vi "Read triangles from stl file (binary format).vi"(0 "STL file path":path=path "C:/EnFlo Software/Anemometry/Anemometry Sub Vis/Collision_Detection/Triangles/Example files/SR-71_Blackbird.STL") -> (1 "Triangles array":T1[](array[typedef]), 2 "N triangles":u32=3528, 3 "Error out":errorcluster)   [LabVIEW 2014]
doc: "Note: The STL file must be in binary format, not ASCII."
uses:
  Typedefs/Triangle.ctl
panel:
  out "STL header":string
  # "PN 19/01/2015"
  # "Vertices"
  # "Edges"
  # "Unit normal"
  # "pre-store"
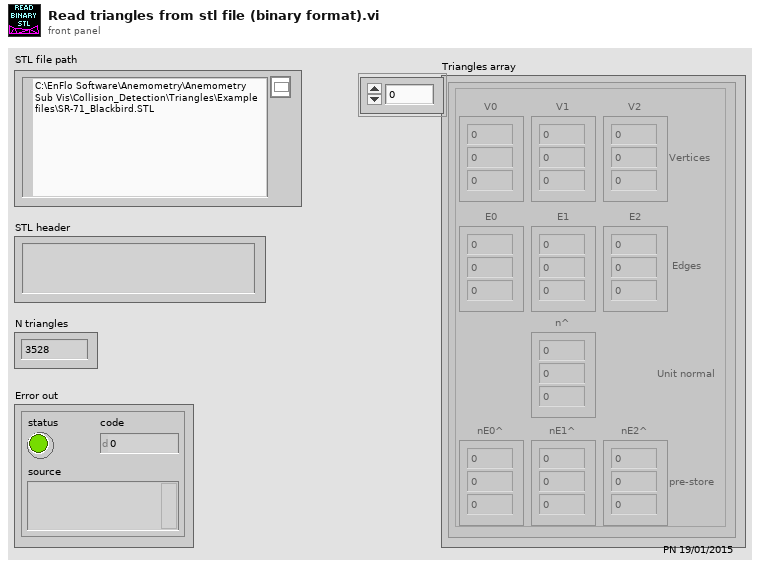
[diagram p1: front panel]
types:
  T1 = typedef "Triangle.ctl" = cluster{"V0":sgl[], "V1":sgl[], "V2":sgl[], "E0":sgl[], "E1":sgl[], "E2":sgl[], "n^":sgl[], "nE0^":sgl[], "nE1^":sgl[], "nE2^":sgl[]}
  T2 = enum16{"big-endian, network order", "native, host order", "little-endian"}
  T3 = enum16{"open", "replace", "create", "open or create", "replace or create", "replace or create with confirmation"}
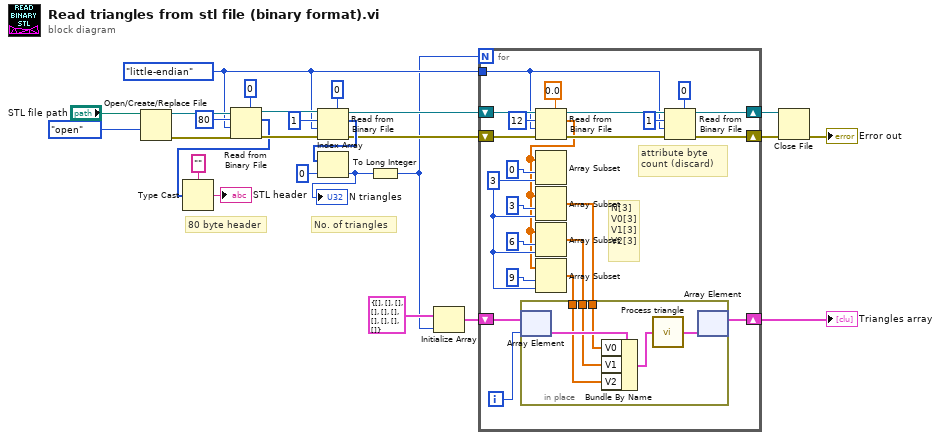
[diagram p0: block diagram]
diagram:
  w3 = T2."little-endian" ("byte order (0:big-endian, network order)")
  # "No. of triangles"
  # "80 byte header"
  n1 = Open/Create/Replace File(file path (use dialog)="STL file path", operation (0:open)=T3."open") -> (refnum out=w24:refnum<file>, error out=w23:errorcluster)  [unwired: 4 in, 1 out]
  n2 = Read from Binary File(5:u8 0, 8:w23, 9:w3, 10:80 ("count (1)"), 11:w24) -> (0:w16:errorcluster, 2:w14:u8[], 3:w18:refnum<file>)  [unwired: 1 in, 1 out]
  n3 = Type Cast(type="", x=w14) -> (*(type *) &x=→"STL header":string)
  n4 = Read from Binary File(5:u32 0, 8:w16, 9:w3, 10:1 ("count (1)"), 11:w18) -> (0:w11:errorcluster, 2:w13:u32[], 3:w10:refnum<file>)  [unwired: 1 in, 1 out]
  n5 = Index Array(array=w13, index=0) -> (element=w12:u32)
  "N triangles" <- w12
  n6 = To Long Integer(number=w12) -> (32bit integer=w2:i32)
  n7 = Initialize Array(T1 {"V0"=[], "V1"=[], "V2"=[], "E0"=[], "E1"=[], "E2"=[], "n^"=[], "nE0^"=[], "nE1^"=[], "nE2^"=[]} ("Cluster"), w2) -> (w5:T1[])
  n8 = for {
    N: w2 -> [_]
    shift-right: [w40] -> w8
    shift-left: w11 -> [w48]
    shift-right: [w41] -> w9
    shift-left: w10 -> [w49]
    shift-right: [w38] -> w1
    shift-left: w5 -> [w39]
    tunnel: w3 -> [w28]
    i -> [w27]
    w33 = 3 ("length")
    # "N[3]\nV0[3]\nV1[3]\nV2[3]"
    # "attribute byte count (discard)"
    n9 = Read from Binary File(5:sgl 0.0, 8:w48, 9:w28, 10:12 ("count (1)"), 11:w49) -> (0:w43:errorcluster, 2:w32:sgl[], 3:w42:refnum<file>)  [unwired: 1 in, 1 out]
    n10 = Array Subset(array=w32, index=0, length=w33) -> ()  [unwired: 1 out]
    n11 = Array Subset(array=w32, index=3, length=w33) -> (w31:sgl[])
    n12 = Array Subset(array=w32, index=6, length=w33) -> (w30:sgl[])
    n13 = Array Subset(array=w32, index=9, length=w33) -> (w29:sgl[])
    n14 = in-place {
      in-place-border: w31 -> [w52]
      in-place-border: w30 -> [w51]
      in-place-border: w29 -> [w50]
      n15 = in-place-array #1(w39, w27) -> (w54:T1)
      n16 = Bundle By Name(cluster=w54, "V0"=w52, "V1"=w51, "V2"=w50) -> (w53:T1)
      n17 = call "Process triangle.vi"("Triangle in"=w53) -> ("Triangle out"=w55:T1)
      n18 = in-place-array #1(w55) -> (w38:T1[])  [unwired: 1 out]
    }
    n19 = Read from Binary File(5:u16 0, 8:w43, 9:w28, 10:1 ("count (1)"), 11:w42) -> (0:w40:errorcluster, 3:w41:refnum<file>)  [unwired: 1 in, 2 out]
  }
  "Triangles array" <- w1
  n20 = Close File(refnum=w9, error in=w8) -> (error out=→"Error out":errorcluster)  [unwired: 1 out]
